vi "CalculateImageSize.vi"(8 "error in (no error)":errorcluster, 10 "String":string, 11 "Code39 in":refnum<class "Code39.lvclass">) -> (0 "error out":errorcluster, 2 "Size":cluster{"x":i16, "y":i16}, 3 "Code39 out":refnum<class "Code39.lvclass">)   [LabVIEW 2013, in "BarCodes.lvlib" / "Code39.lvclass"]
doc: "Calculates the size of the image for the barcode. This should include the entire barcode, quiet space, and text around it."
uses:
  Code39.lvclass
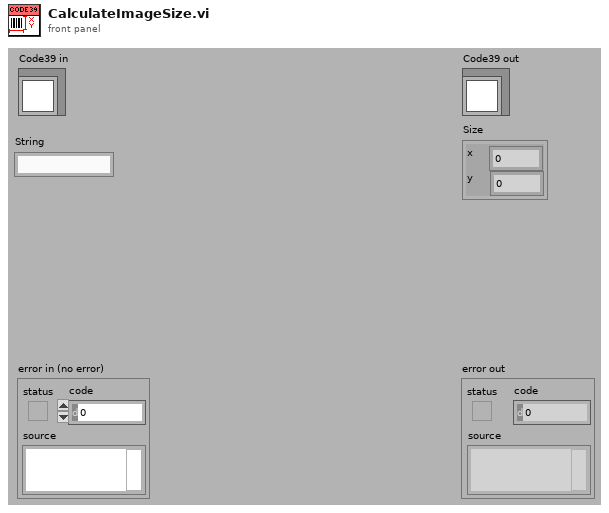
[diagram p1: front panel]
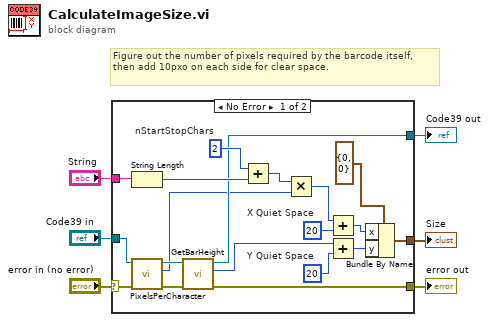
[diagram p0: block diagram]
diagram:
  # "Figure out the number of pixels required by the barcode itself, then add 10pxo on each side for clear space."
  n1 = case shown="No Error" "error in (no error)" {
    selector: "error in (no error)" -> [w7 w26]
    tunnel: "String" -> [w25 _]
    tunnel: [w17 w27] -> w5
    tunnel: [w16 w26] -> w4
    tunnel: [w12 _] -> w3
    tunnel: "Code39 in" -> [w11 w27]
    frame No Error {
      w14 = 20  # Y Quiet Space
      w20 = 20  # X Quiet Space
      w23 = 2  # nStartStopChars
      n2 = String Length(string=w25) -> (length=w24:i32)
      n3 = call "PixelsPerCharacter.vi"("error in (no error)"=w7, "Code39 in"=w11) -> ("error out"=w10:errorcluster, "Pixels per Character"=w8:u8, "Code39 out"=w9:refnum<class "Code39.lvclass">)  [unwired: 7 in]
      n4 = call-dynamic "GetBarHeight.vi"("error in (no error)"=w10, "Code39 in"=w9) -> ("error out"=w16:errorcluster, "Bar Height"=w15:u8, "Code39 out"=w17:refnum<class "Code39.lvclass">)  [unwired: 7 in]
      n5 = Add(x=w23, y=w24) -> (x+y=w22:i32)
      n6 = Multiply(x=w22, y=w8) -> (x*y=w21:i32)
      n7 = Add(x=w21, y=w20) -> (x+y=w18:i32)
      n8 = Add(x=w15, y=w14) -> (x+y=w13:i32)
      n9 = Bundle By Name(cluster=cluster{"x":i16, "y":i16} {"x"=0, "y"=0} ("Size"), "x"=w18, "y"=w13) -> (w12:cluster{"x":i16, "y":i16})
    }
    frame Error {
    }
  }
  "error out" <- w4
  "Code39 out" <- w5
  "Size" <- w3
